vi "loadDataToBuffer.vi"(8 "error in (no error)":errorcluster, 11 "HamegHMPSupply in":refnum<class "HamegHMPSupply.lvclass">) -> (0 "error out":errorcluster, 3 "HamegHMPSupply out":refnum<class "HamegHMPSupply.lvclass">)   [LabVIEW 2011, in "Hardware.lvlib" / "Channels.lvlib" / "HamegHMPSupply.lvclass"]
doc: "Abstract Method.\n\nThis vi, via its implementing classes, loads the analog output data to the buffer of the device."
uses:
  HamegHMPSupply.lvclass
  HamegHMPSupply.lvclass/HamegHMPSupply.ctl
  AnalogOutput.lvclass
panel:
  out "Data":dbl[][](array[numeric])
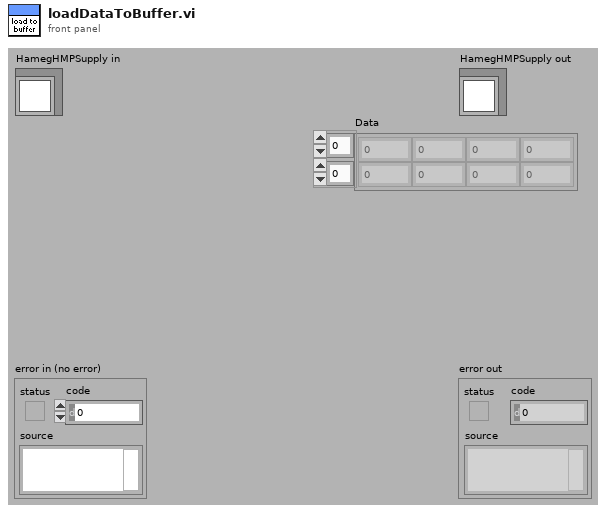
[diagram p1: front panel]
types:
  T1 = cluster{"VoltageLimit":dbl, "CurrentLimit":dbl}[]
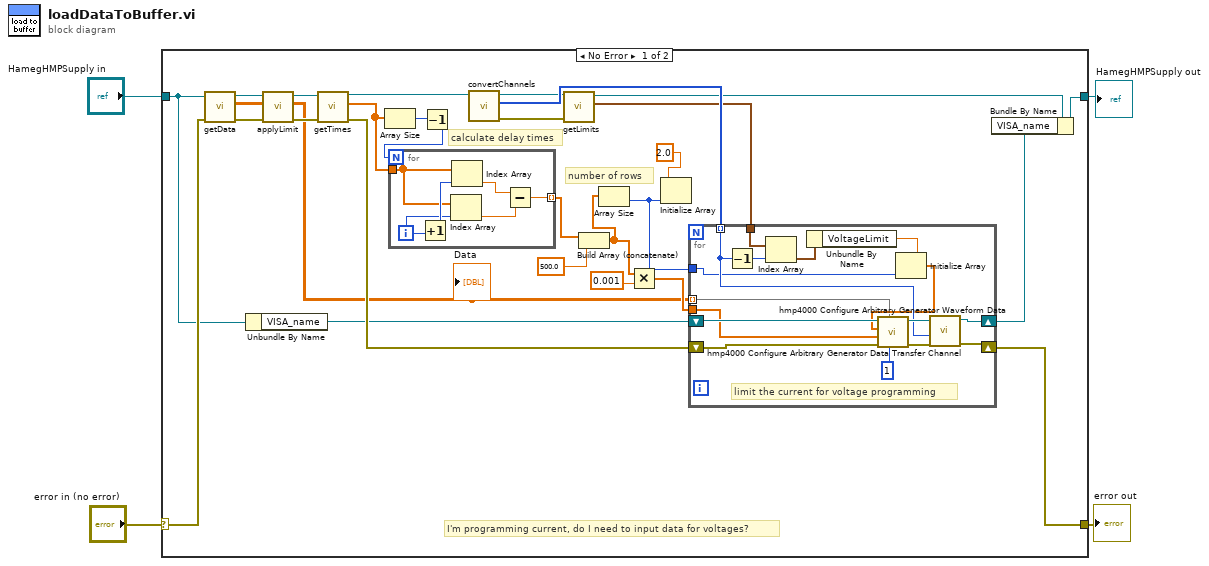
[diagram p0: block diagram]
diagram:
  n1 = case shown="No Error" "error in (no error)" {
    selector: "error in (no error)" -> [w33 w56]
    tunnel: "HamegHMPSupply in" -> [w30 w57]
    tunnel: [w29 w57] -> w2
    tunnel: [w32 w56] -> w1
    frame No Error {
      # "number of rows"
      # "I'm programming current, do I need to input data for voltages?"
      # "calculate delay times"
      n2 = call "getData.vi"("error in (no error)"=w33, "AnalogOutput.lvclass in"=w30) -> ("error out"=w6:errorcluster, "Data"=w10:dbl[][], "AnalogOutput.lvclass out"=w9:refnum<class "HamegHMPSupply.lvclass">)  [unwired: 7 in]
      n3 = Unbundle By Name(w30) -> ("VISA_name"=w19:refnum<visa-resource-name>)
      n4 = call "applyLimit.vi"("error in (no error)"=w6, "Data"=w10, "HamegHMPSupply in"=w9) -> ("error out"=w7:errorcluster, "Data"=w5:dbl[][], "HamegHMPSupply out"=w8:refnum<class "HamegHMPSupply.lvclass">)  [unwired: 6 in]
      "Data" <- w5
      n5 = call "getTimes.vi"("error in (no error)"=w7, "AnalogOutput in"=w8) -> ("error out"=w31:errorcluster, "times"=w27:dbl[], "AnalogOutput out"=w24:refnum<class "HamegHMPSupply.lvclass">)  [unwired: 7 in]
      n6 = Array Size(array=w27) -> (size(s)=w26:i32)
      n7 = Decrement(x=w26) -> (x-1=w25:i32)
      n8 = for {
        N: w25 -> [_]
        tunnel: w27 -> [w51]
        tunnel: [w53] -> w21 mode=indexing
        i -> [w50]
        n9 = Increment(x=w50) -> (x+1=w55:i32)
        n10 = Index Array(array=w51, index=w50) -> (element=w52:dbl)
        n11 = Index Array(array=w51, index=w55) -> (element=w54:dbl)
        n12 = Subtract(x=w54, y=w52) -> (x-y=w53:dbl)
      }
      n13 = call "convertChannels.vi"("HamegHMPSupply in"=w24) -> ("error out"=w14:errorcluster, "channels"=w23:i32[], "HamegHMPSupply out"=w15:refnum<class "HamegHMPSupply.lvclass">)  [unwired: 8 in]
      n14 = call "getLimits.vi"("error in (no error)"=w14, "AnalogOutput in"=w15) -> ("Limits"=w12:T1, "AnalogOutput out"=w13:refnum<class "HamegHMPSupply.lvclass">)  [unwired: 7 in, 1 out]
      n15 = Build Array (concatenate)(w21, 500.0) -> (w18:dbl[])
      n16 = Array Size(array=w18) -> (size(s)=w11:i32)
      n17 = Multiply(x=w18, y=0.001) -> (x*y=w16:dbl[])
      n18 = Initialize Array(2.0, w11) -> ()  [unwired: 1 out]
      n19 = for {
        shift-right: [w43] -> w32
        shift-left: w31 -> [w47]
        shift-right: [w45] -> w28
        shift-left: w19 -> [w48]
        tunnel: w5 -> [w34] mode=indexing
        tunnel: w16 -> [w36]
        tunnel: w23 -> [w41] mode=indexing
        tunnel: w12 -> [w42]
        tunnel: w11 -> [w37]
        # "limit the current for voltage programming"
        n20 = Decrement(x=w41) -> (x-1=w40:i32)
        n21 = Index Array(array=w42, index=w40) -> (element=w39:cluster{"VoltageLimit":dbl, "CurrentLimit":dbl})
        n22 = Unbundle By Name(w39) -> ("VoltageLimit"=w38:dbl)
        n23 = Initialize Array(w38, w37) -> (w35:dbl[])
        n24 = call <instrlib>:"hmp4000 Configure Arbitrary Generator Waveform Data.vi"("Repetition (0)"=1, "Current"=w34, "error in (no error)"=w47, "Time"=w36, "Voltage"=w35, "VISA resource name"=w48) -> ("error out"=w44:errorcluster, "VISA resource name out"=w46:refnum<visa-resource-name>)  [unwired: 4 in]
        n25 = call <instrlib>:"hmp4000 Configure Arbitrary Generator Data Transfer Channel.vi"("error in (no error)"=w44, "Channel (Channel 1)"=w41, "VISA resource name"=w46) -> ("error out"=w43:errorcluster, "VISA resource name out"=w45:refnum<visa-resource-name>)  [unwired: 7 in]
      }
      n26 = Bundle By Name(cluster=w13, "VISA_name"=w28) -> (w29:refnum<class "HamegHMPSupply.lvclass">)
    }
    frame Error {
    }
  }
  "error out" <- w1
  "HamegHMPSupply out" <- w2
